vi "Read ADU Packet.vi"(8 "error in":errorcluster, 10 "protocol layer":refnum<class "Network Protocol.lvclass">, 11 "IP transmission data unit in":refnum<class "IP Data Unit.lvclass">) -> (0 "error out":errorcluster, 1 "modbus data unit":refnum<class "Modbus Data Unit.lvclass">, 2 "protocol layer out":refnum<class "Network Protocol.lvclass">, 3 "IP transmission data unit out":refnum<class "IP Data Unit.lvclass">, 5 "PDU Valid?":bool)   [LabVIEW 2013, in "Modbus Library - Advance.lvlib" / "IP Data Unit.lvclass"]
doc: "This uses the protocol layer to read a modbus packet off of the bus, wrapped in the IP transmission data unit."
uses:
  IP Data Unit.lvclass
  Modbus Data Unit/Modbus Data Unit.lvclass
  Network Protocol/Network Protocol.lvclass
  Transmission Data Unit.lvclass/Transmission Data Unit.ctl
  IP Data Unit.lvclass/IP Data Unit.ctl
  Modbus Data Unit/Modbus Data Unit.lvclass/Modbus Data Unit.ctl
  <vilib>/Utility/error.llb/Error Cluster From Error Code.vi
  <vilib>/ErrorRing/Error Ring.xnode
  Transmission Data Unit.lvclass
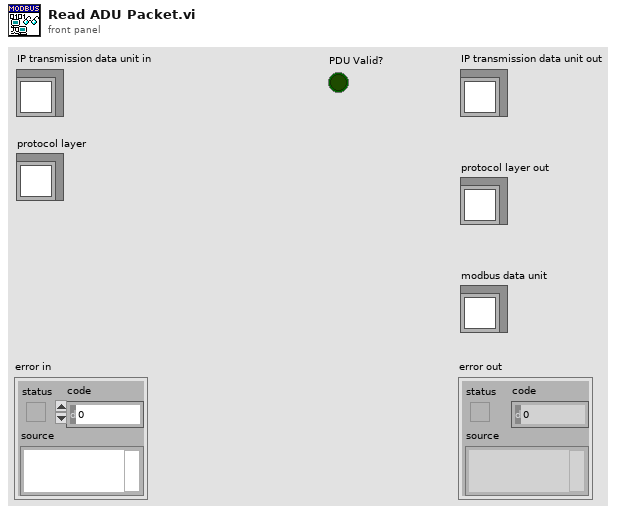
[diagram p1: front panel]
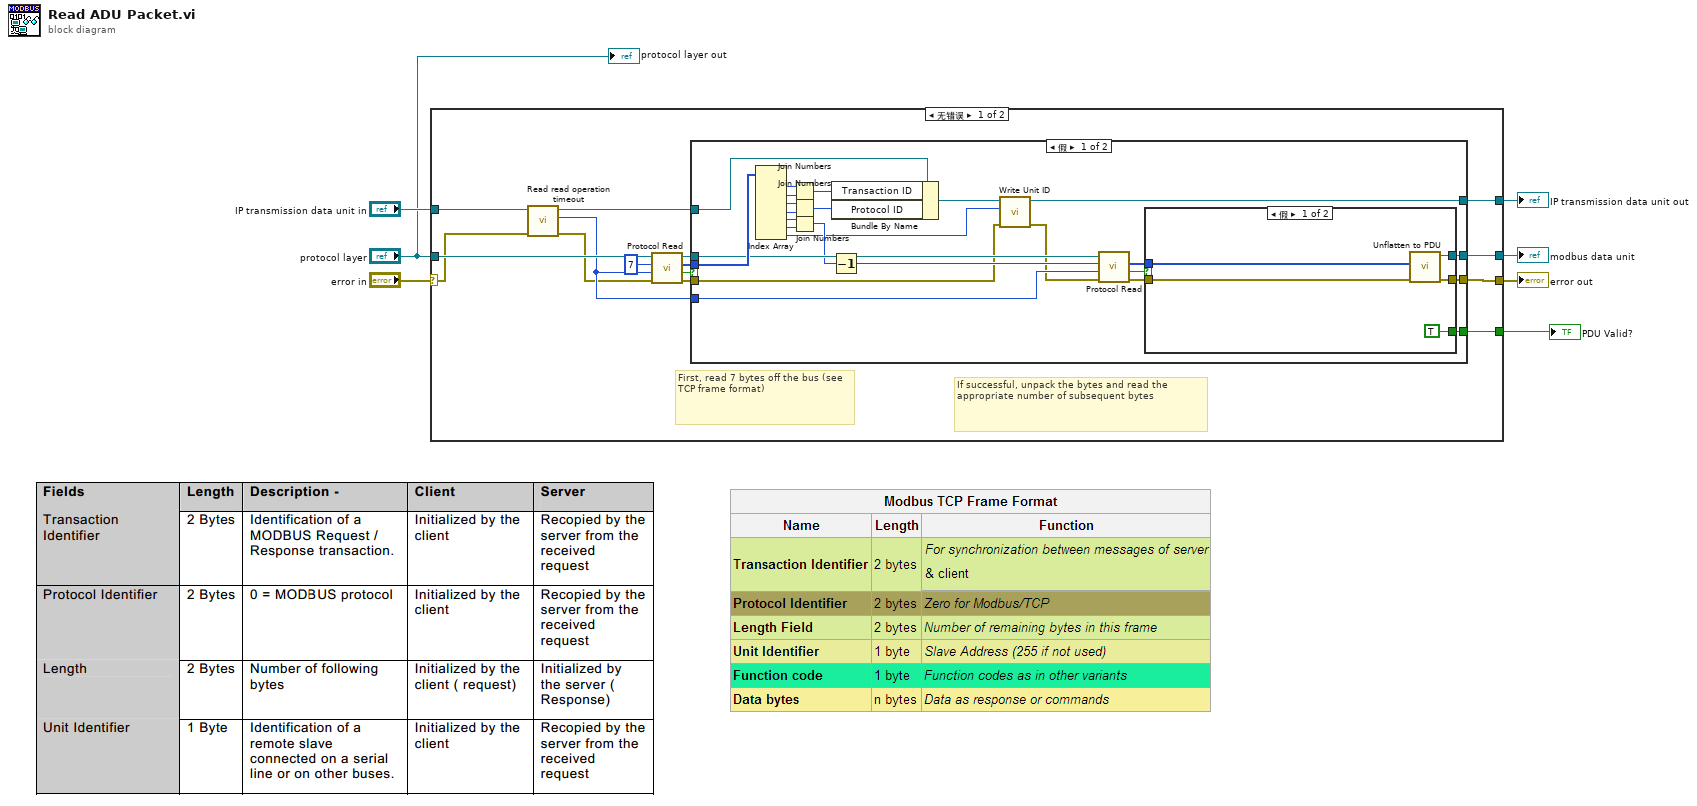
[diagram p0: block diagram]
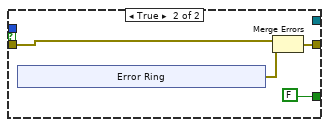
[diagram p2: hidden frame]
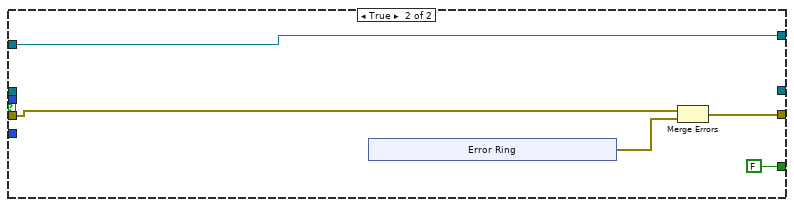
[diagram p3: hidden frame]
diagram:
  n1 = case shown="无错误" "error in" {
    selector: "error in" -> [w8 w71]
    tunnel: [w16 w71] -> w6
    tunnel: "IP transmission data unit in" -> [w9 w70]
    tunnel: [w19 w70] -> w4
    tunnel: "protocol layer" -> [w22 _]
    tunnel: [w15 _] -> w3
    tunnel: [w10 _] -> w1
    frame No Error {
      # "If successful, unpack the bytes and read the appropriate number of subsequent bytes"
      # "First, read 7 bytes off the bus (see TCP frame format)"
      n2 = call "Read read operation timeout.vi"("error in (no error)"=w8, "transmission data unit in"=w9) -> ("error out"=w11:errorcluster, "read operation timeout"=w13:i32, "transmission data unit out"=w12:refnum<class "IP Data Unit.lvclass">)  [unwired: 7 in]
      n3 = call-dynamic "Protocol Read.vi"("error in"=w11, "timeout"=w13, "bytes to read"=7 ("Bytes to Read"), "protocol layer in"=w22) -> ("error out"=w17:errorcluster, "timed out?"=w14:bool, "data"=w20:u8[], "protocol layer out"=w18:refnum<class "Network Protocol.lvclass">)  [unwired: 4 in]
      n4 = case shown="假" w14 {
        tunnel: w20 -> [w47 _]
        tunnel: w12 -> [w46 w65]
        tunnel: [w27 w65] -> w19
        tunnel: w18 -> [w37 _]
        tunnel: w13 -> [w35 _]
        tunnel: w17 -> [w25 w62]
        tunnel: [w32 w63] -> w16
        tunnel: [w31 _] -> w15
        tunnel: [w24 FALSE] -> w10
        frame False {
          n5 = Index Array(array=w47) -> (element #1=w44:u8, element #2=w45:u8, element #3=w42:u8, element #4=w41:u8, element #5=w38:u8, element #6=w39:u8, element #7=w23:u8)  [unwired: 7 in]
          n6 = Join Numbers(hi=w44, lo=w45) -> ((hi.lo)=w43:u16)
          n7 = Join Numbers(hi=w42, lo=w41) -> ((hi.lo)=w40:u16)
          n8 = Join Numbers(hi=w38, lo=w39) -> ((hi.lo)=w36:u16)
          n9 = Decrement(x=w36) -> (x-1=w34:u16)
          n10 = Bundle By Name(cluster=w46, "Transaction ID"=w43, "Protocol ID"=w40) -> (w28:refnum<class "IP Data Unit.lvclass">)
          n11 = call "Write Unit ID.vi"("error in"=w25, "unit ID"=w23, "transmission data unit in"=w28) -> ("error out"=w26:errorcluster, "transmission data unit out"=w27:refnum<class "IP Data Unit.lvclass">)  [unwired: 7 in]
          n12 = call-dynamic "Protocol Read.vi"("error in"=w26, "timeout"=w35, "bytes to read"=w34, "protocol layer in"=w37) -> ("error out"=w33:errorcluster, "timed out?"=w29:bool, "data"=w30:u8[])  [unwired: 4 in, 1 out]
          n13 = case shown="假" w29 {
            tunnel: w33 -> [w52 w55]
            tunnel: [w51 w56] -> w32
            tunnel: [w50 _] -> w31
            tunnel: w30 -> [w49 _]
            tunnel: [TRUE FALSE] -> w24
            frame False {
              n14 = call "Unflatten to PDU.vi"("error in"=w52, "modbus data unit data"=w49) -> ("error out"=w51:errorcluster, "modbus data unit out"=w50:refnum<class "Modbus Data Unit.lvclass">)  [unwired: 8 in]
            }
            frame True {
              n15 = xnode "Error Ring"() -> ("错误输出"=w54:errorcluster)
              n16 = Merge Errors(w55, w54) -> (w56:errorcluster)
            }
          }
        }
        frame True {
          n17 = xnode "Error Ring"() -> ("错误输出"=w64:errorcluster)
          n18 = Merge Errors(w62, w64) -> (w63:errorcluster)
        }
      }
    }
    frame Error {
    }
  }
  "error out" <- w6
  "IP transmission data unit out" <- w4
  "modbus data unit" <- w3
  "PDU Valid?" <- w1
  "protocol layer out" <- "protocol layer"
